vi "Calculate Total Ramp Period Power Down.vi"(5 "Relative To":T1[](array[typedef]) items=["Power sequence start", "Previous source start", "Previous source end"], 7 "Level":dbl[](array[numeric]), 9 "Ramp Rate":dbl[](array[numeric]), 11 "Sequence Delta":dbl[](array[numeric])) -> (6 "Total Power Seq Period":dbl format="%#_6p", 8 "Idle Time after ramp":dbl[](array[numeric]) format="%#_6p")   [LabVIEW 2024, in "devicePowerSequencerCoreLogic.lvlib"]
uses:
  devicePowerSequencerCoreLogic.lvlib
  controls/Relative To.ctl
  devicePowerSequencer.lvlib
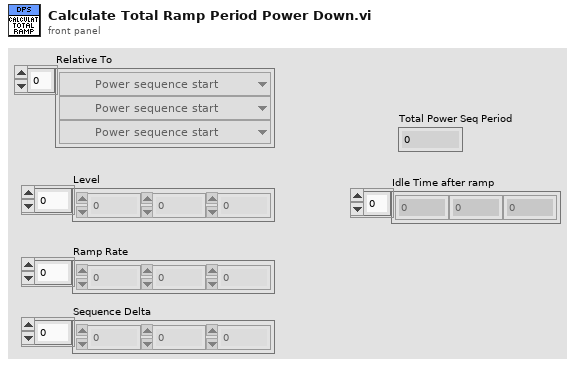
[diagram p1: front panel]
types:
  T1 = typedef "devicePowerSequencer.lvlib/Relative To.ctl" = u32
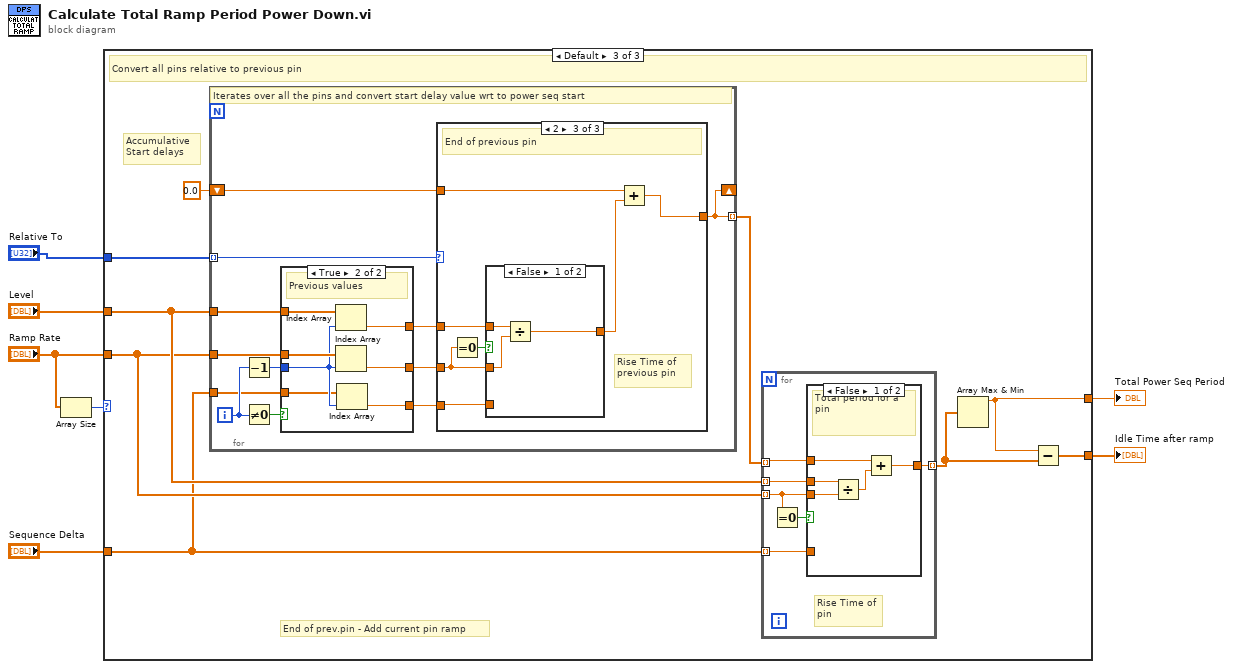
[diagram p0: block diagram]
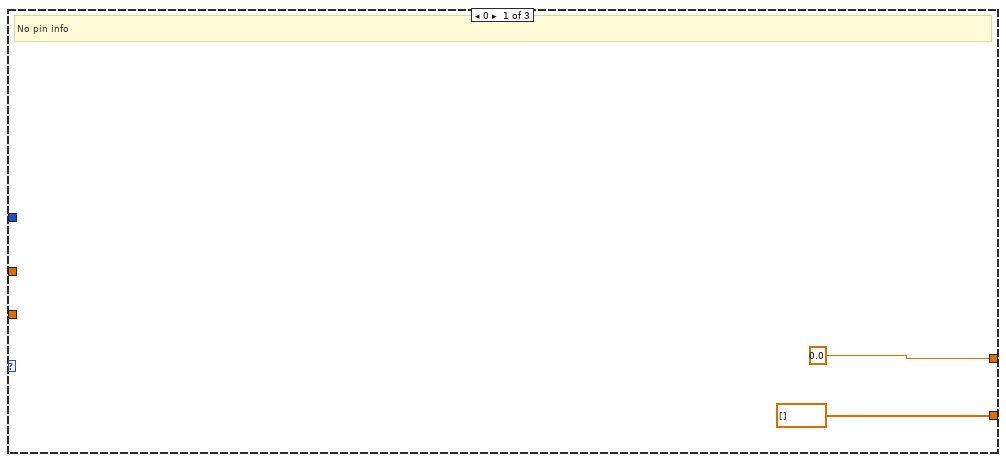
[diagram p2: hidden frame]
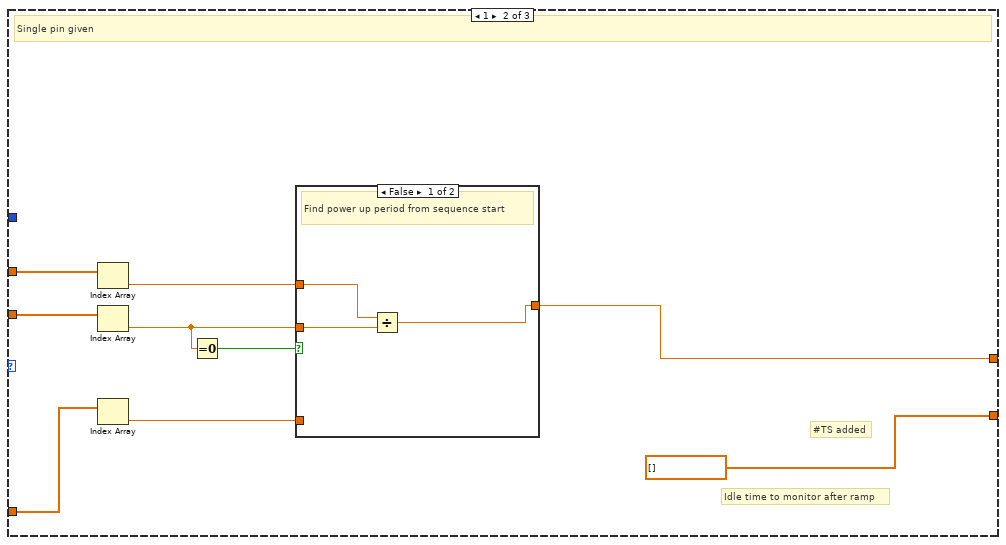
[diagram p3: hidden frame]
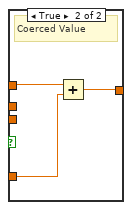
[diagram p5: hidden frame]
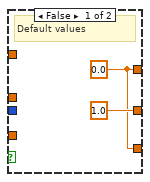
[diagram p6: hidden frame]
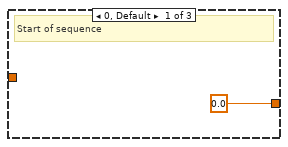
[diagram p7: hidden frame]
diagram:
  n1 = Array Size(array="Ramp Rate") -> (size(s)=w4:i32)
  n2 = case shown="Default" w4 {
    tunnel: "Relative To" -> [_ _ w31]
    tunnel: "Level" -> [_ w18 w29]
    tunnel: "Ramp Rate" -> [_ w17 w28]
    tunnel: [0.0 w16 w24] -> w6
    tunnel: [dbl[] [] dbl[] [] w26] -> w3
    tunnel: "Sequence Delta" -> [_ w12 w23]
    frame 0 {
      # "No pin info"
    }
    frame 1 {
      # "#TS added"
      # "Idle time to monitor after ramp"
      # "Single pin given"
      n3 = Index Array(array=w18) -> (element=w13:dbl)  [unwired: 1 in]
      n4 = Index Array(array=w17) -> (element=w14:dbl)  [unwired: 1 in]
      n5 = Index Array(array=w12) -> (element=w11:dbl)  [unwired: 1 in]
      n6 = Equal To 0?(x=w14) -> (x = 0?=w10:bool)
      n7 = case shown="False" w10 {
        tunnel: [w21 w22] -> w16
        tunnel: w14 -> [w20 _]
        tunnel: w13 -> [w19 _]
        tunnel: w11 -> [_ w22]
        frame False {
          # "Find power up period from sequence start"
          n8 = Divide(x=w19, y=w20) -> (x/y=w21:dbl)
        }
        frame True {
          # "Default Ramp Rate"
        }
      }
    }
    frame Default {
      # "End of prev.pin - Add current pin ramp"
      # "Accumulative\nStart delays"
      # "Convert all pins relative to previous pin"
      n9 = for {
        tunnel: w31 -> [w57] mode=indexing
        tunnel: w28 -> [w53]
        tunnel: [w52] -> w27 mode=indexing
        shift-right: [w52] -> _
        shift-left: 0.0 ("Numeric") -> [w56]
        tunnel: w29 -> [w54]
        tunnel: w23 -> [w47]
        i -> [w51]
        # "Iterates over all the pins and convert start delay value wrt to power seq start"
        n10 = Decrement(x=w51) -> (x-1=w50:i32)
        n11 = Not Equal To 0?(x=w51) -> (x != 0?=w55:bool)
        n12 = case shown="True" w55 {
          tunnel: w54 -> [_ w66]
          tunnel: w53 -> [_ w65]
          tunnel: w50 -> [_ w62]
          tunnel: [w58 w64] -> w49
          tunnel: [1.0 ("Numeric") w63] -> w48
          tunnel: w47 -> [_ w61]
          tunnel: [w58 w60] -> w46
          frame False {
            w58 = 0.0 ("Numeric")
            # "Default values"
          }
          frame True {
            # "Previous values"
            n13 = Index Array(array=w66, index=w62) -> (element=w64:dbl)
            n14 = Index Array(array=w65, index=w62) -> (element=w63:dbl)
            n15 = Index Array(array=w61, index=w62) -> (element=w60:dbl)
          }
        }
        n16 = case shown="2" w57 {
          tunnel: [0.0 w68 w69] -> w52
          tunnel: w56 -> [_ w68 w75]
          tunnel: w49 -> [_ _ w73]
          tunnel: w48 -> [_ _ w71]
          tunnel: w46 -> [_ _ w70]
          frame 0, Default {
            # "Start of sequence"
          }
          frame 1 {
            # "Start of previous pin"
          }
          frame 2 {
            # "Rise Time of previous pin"
            # "End of previous pin"
            n17 = Equal To 0?(x=w71) -> (x = 0?=w72:bool)
            n18 = case shown="False" w72 {
              tunnel: [w78 w79] -> w74
              tunnel: w73 -> [w77 _]
              tunnel: w71 -> [w76 _]
              tunnel: w70 -> [_ w79]
              frame False {
                n19 = Divide(x=w77, y=w76) -> (x/y=w78:dbl)
              }
              frame True {
                # "Single step dt is considered when ramp rate control is not defined"
              }
            }
            n20 = Add(x=w75, y=w74) -> (x+y=w69:dbl)
          }
        }
      }
      n21 = for {
        tunnel: w29 -> [w37] mode=indexing
        tunnel: w28 -> [w34] mode=indexing
        tunnel: w27 -> [w36] mode=indexing
        tunnel: [w35] -> w25 mode=indexing
        tunnel: w23 -> [w32] mode=indexing
        # "Rise Time of pin"
        n22 = Equal To 0?(x=w34) -> (x = 0?=w33:bool)
        n23 = case shown="False" w33 {
          tunnel: w37 -> [w42 _]
          tunnel: w34 -> [w41 _]
          tunnel: w36 -> [w40 w45]
          tunnel: [w38 w43] -> w35
          tunnel: w32 -> [_ w44]
          frame False {
            # "Total period for a pin"
            n24 = Divide(x=w42, y=w41) -> (x/y=w39:dbl)
            n25 = Add(x=w40, y=w39) -> (x+y=w38:dbl)
          }
          frame True {
            # "Coerced Value"
            n26 = Add(x=w45, y=w44) -> (x+y=w43:dbl)
          }
        }
      }
      n27 = Array Max & Min(array=w25) -> (max value=w24:dbl)  [unwired: 3 out]
      n28 = Subtract(x=w24, y=w25) -> (x-y=w26:dbl[])
    }
  }
  "Total Power Seq Period" <- w6
  "Idle Time after ramp" <- w3
